vi "Ctor.vi"(8 "error in (no error)":errorcluster, 11 "PropertyObject in":refnum<class "PropertyObject.lvclass">) -> (0 "error out":errorcluster, 3 "PropertyObject out":refnum<class "PropertyObject.lvclass">)   [LabVIEW 2020, in "TSnax.lvlib" / "PropertyObject.lvclass"]
uses:
  PropertyObject.lvclass
  Ref Data.ctl
  PropertyObject.lvclass/PropertyObject.ctl
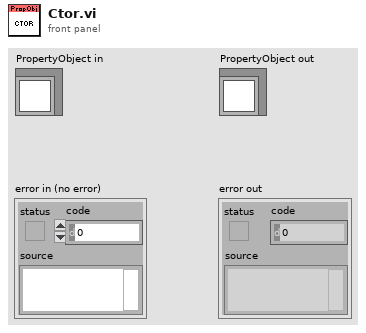
[diagram p1: front panel]
types:
  T1 = typedef "TSnax.lvlib/PropertyObject.lvclass/Ref Data.ctl" = cluster{"PropertyObject":refnum<k7>}
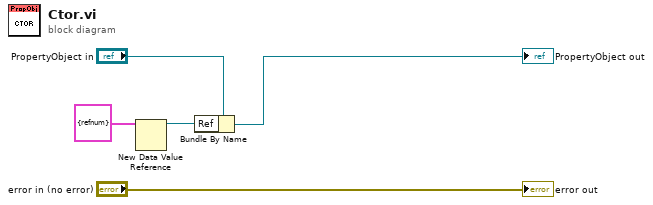
[diagram p0: block diagram]
diagram:
  n1 = New Data Value Reference(data value=T1 {"PropertyObject"=refnum} ("Ref Data")) -> (data value reference=w1:refnum<data-value>)  [unwired: 1 in, 1 out]
  n2 = Bundle By Name(cluster="PropertyObject in", "Ref"=w1) -> (→"PropertyObject out":refnum<class "PropertyObject.lvclass">)
  "error out" <- "error in (no error)"
